vi "save HRT data.vi"(9 "coagulant dose":dbl, 10 "Coagulant":T1={"flocculator volume (L)"=100.0, "clarifier volume (L)"=0.0, "dose updates per HRT"=0, "target clarified turbidity (NTU)"=0.3, "Coagulant mode"=enum."manual", "Coag dose [mg/L]"=0.0, "pump mL/rev"=0.0, "clarifier flow [L/s]"=0.5, "min Coag dose [mg/L]"=0.0, "max Coag dose [mg/L]"=0.0, "Steps"=3, "HRT response delay"=1, "Ku*"=1.0} {"HRT response delay" min=1 max=10 step=1; "Steps" min=3 step=1; "clarifier flow [L/s]" min=0.0001 max=1.0 step=0.0001; "target clarified turbidity (NTU)" min=0.1 max=5.0 step=0.01; "dose updates per HRT" min=1 max=100 step=1}) -> ()   [LabVIEW 2015]
uses:
  Sensor buffer command.ctl
  coag.ctl
  model type.ctl
panel:
  out "data labels":string[](array[string])
  # "min"
  # "max"
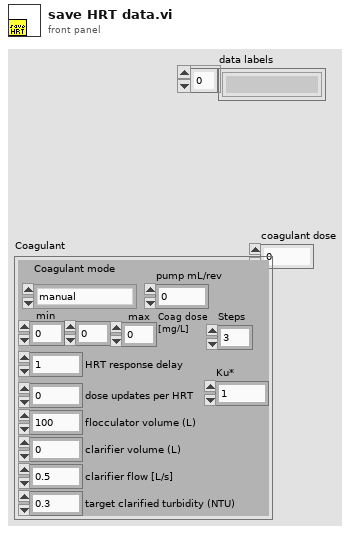
[diagram p1: front panel]
types:
  T1 = typedef "coag.ctl" = cluster{"flocculator volume (L)":dbl, "clarifier volume (L)":dbl, "dose updates per HRT":u16, "target clarified turbidity (NTU)":dbl, "Coagulant mode":T2, "Coag dose [mg/L]":dbl, "pump mL/rev":dbl, "clarifier flow [L/s]":dbl, "min Coag dose [mg/L]":dbl, "max Coag dose [mg/L]":dbl, "Steps":u16, "HRT response delay":u32, "Ku*":dbl}
  T2 = typedef "model type.ctl" = enum16{"manual", "ramp", "simple corrector", "linear regression"}
  T3 = typedef "Sensor buffer command.ctl" = enum16{"set buffer size", "write", "refill buffer", "read recent", "read all", "clear"}
  T4 = typedef "data cluster.ctl" = cluster{"floc sed turbidity (NTU)":dbl, "Raw turbidity (NTU)":dbl, "flow rate (L/s)":dbl, "time":timestamp}
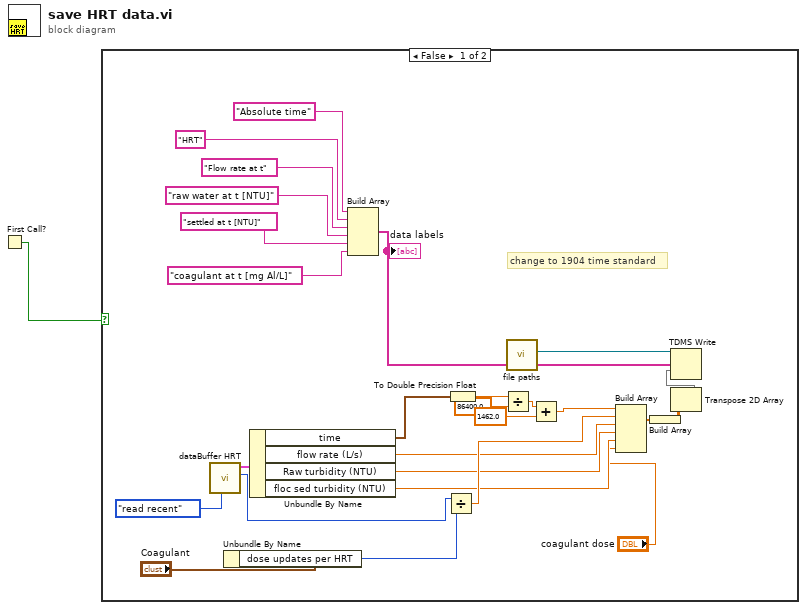
[diagram p0: block diagram]
diagram:
  n1 = First Call?() -> (First Call?: T/F=w1:bool)
  n2 = case shown="False" w1 {
    frame False {
      # "change to 1904 time standard"
      n3 = call "dataBuffer HRT.vi"("command"=Sensor_buffer_command."read recent") -> ("scans"=w10:i32, "recent data"=w13:T4)  [unwired: 7 in, 2 out]
      n4 = Unbundle By Name("Coagulant") -> ("dose updates per HRT"=w9:u16)
      n5 = Unbundle By Name(w13) -> ("time"=w11:timestamp, "flow rate (L/s)"=w6:dbl, "Raw turbidity (NTU)"=w5:dbl, "floc sed turbidity (NTU)"=w4:dbl)
      n6 = Build Array("Absolute time", "HRT", "Flow rate at t", "raw water at t [NTU]", "settled at t [NTU]", "coagulant at t [mg Al/L]" ("element")) -> (w24:string[])
      "data labels" <- w24
      n7 = Divide(x=w10, y=w9) -> (x/y=w8:dbl)
      n8 = To Double Precision Float(number=w11) -> (double precision float=w20:dbl)
      n9 = Divide(x=w20, y=86400.0) -> (x/y=w18:dbl)
      n10 = call "file paths.vi"() -> ("coaglog"=w15:refnum<k34>)  [unwired: 8 in, 3 out]
      n11 = Add(x=w18, y=1462.0) -> (x+y=w16:dbl)
      n12 = Build Array(w16, w8, w6, w5, w4, "coagulant dose") -> (w23:dbl[])
      n13 = Build Array(w23) -> (w22:dbl[][])
      n14 = Transpose 2D Array(2D array=w22) -> (transposed array=w21:dbl[][])
      n15 = TDMS Write(0:w15, 7:w24, 9:w21) -> ()  [unwired: 3 in, 4 out]
    }
    frame True {
    }
  }
